vi "BytetoArray.vi"(0 "file path":path, 1 "Ring":u16(ring) items=["midband", "slope", "intercept"], 2 "Range Params":T1={"mb max"=-20.0, "mb min"=-70.0, "slope max"=8.0, "slope min"=-8.0, "int max"=5.0, "int min"=-85.0} {"int min" format="%.2f"; "int max" format="%.2f"; "slope min" format="%.2f"; "slope max" format="%.2f"; "mb min" format="%.2f"; "mb max" format="%.2f"}, 3 "pixels in x":i32=256, 4 "max scale value":i16=243, 5 "pixels in y":i32=240) -> (6 "Raw data":u8[][](array[numeric]), 7 "Scaled data":dbl[][](array[numeric]) format="%.2f", 8 "true orientation":u8[][](array[numeric]))   [LabVIEW 2022 SP3]
panel:
  # "This is prostate format default"
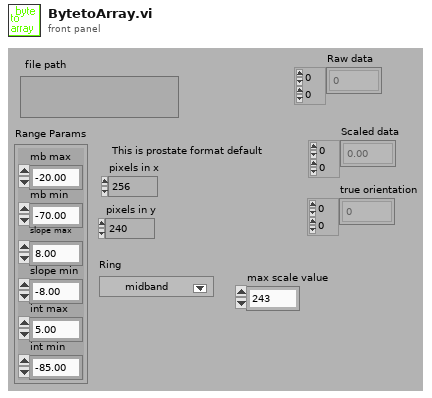
[diagram p1: front panel]
types:
  T1 = cluster{"mb max":dbl, "mb min":dbl, "slope max":dbl, "slope min":dbl, "int max":dbl, "int min":dbl}
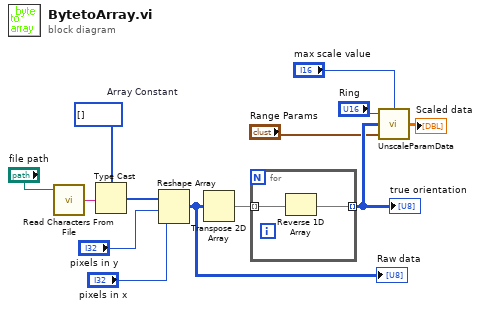
[diagram p0: block diagram]
diagram:
  w12 = u8[] []  # Array Constant
  n1 = call <vilib>:"Read Characters From File.vi"("file path (dialog if empty)"="file path") -> ("character string"=w13:string)  [unwired: 1 in, 7 out]
  n2 = Type Cast(type=w12, x=w13) -> (*(type *) &x=w11:u8[])
  n3 = Reshape Array(w11, "pixels in y", "pixels in x") -> (w8:u8[][])
  "Raw data" <- w8
  n4 = Transpose 2D Array(2D array=w8) -> (transposed array=w9:u8[][])
  n5 = for {
    tunnel: w9 -> [w15] mode=indexing
    tunnel: [w14] -> w5 mode=indexing
    n6 = Reverse 1D Array(array=w15) -> (reversed array=w14:u8[])
  }
  "true orientation" <- w5
  n7 = call "UnscaleParamData.vi"("max scale value"="max scale value", "Range Params"="Range Params", "scaled data"=w5, "Ring"="Ring") -> ("UnScaled data"=→"Scaled data":dbl[][])
